vi "Albert_Arr_QueryString.vi"(10 "字符串":string, 11 "2D Arr Input":string[][](array[string])) -> (3 "2D Arr Output":string[][](array[string]))   [LabVIEW 2018]
panel:
  out "数值":i32
  out "布尔":bool=TRUE
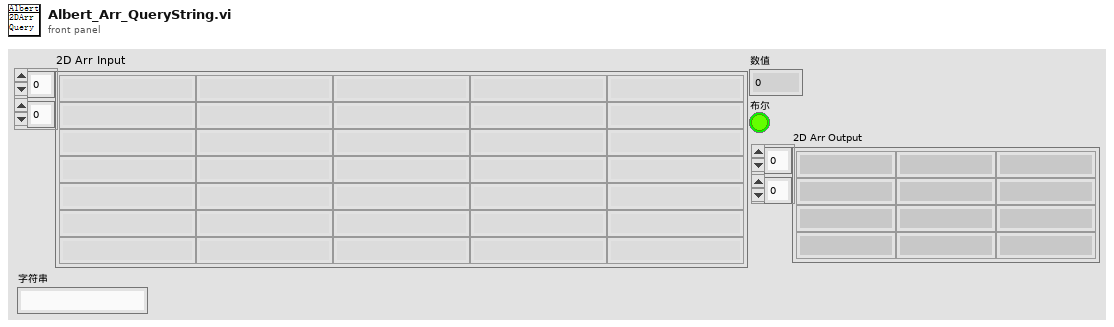
[diagram p1: front panel]
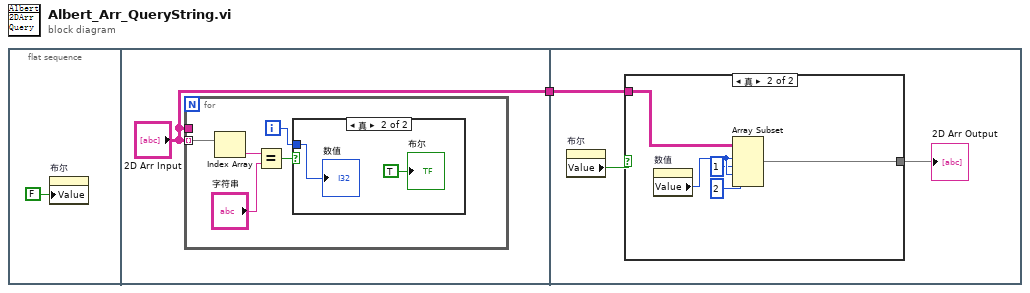
[diagram p0: block diagram]
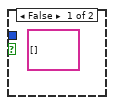
[diagram p2: hidden frame]
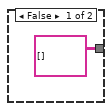
[diagram p3: hidden frame]
diagram:
  n1 = flat-sequence {
    tunnel: ["2D Arr Input"] -> w1
    tunnel: w1 -> [w13]
    frame #0 {
      n2 = property on="布尔" class="Bool (严格)"("Value"=FALSE ("布尔")) -> ()  [unwired: 2 in, 2 out]
    }
    frame #1 {
      n3 = for {
        tunnel: "2D Arr Input" -> [w8] mode=indexing
        tunnel: "2D Arr Input" -> [_]
        i -> [w4]
        n4 = Index Array(array=w8) -> (element=w7:string)  [unwired: 1 in]
        n5 = Equal?(x=w7, y="字符串") -> (x = y?=w5:bool)
        n6 = case shown="真" w5 {
          tunnel: w4 -> [_ w10]
          frame False {
            (unwired) string[][] []
          }
          frame True {
            "数值" <- w10
            "布尔" <- TRUE
          }
        }
      }
    }
    frame #2 {
      n7 = property on="布尔" class="Bool (严格)"() -> ("Value"=w12:bool)  [unwired: 2 in, 2 out]
      n8 = case shown="真" w12 {
        tunnel: w13 -> [_ w19]
        tunnel: [string[][] [] w15] -> w11
        frame False {
        }
        frame True {
          n9 = property on="数值" class="DigNum (严格)"() -> ("Value"=w18:i32)  [unwired: 2 in, 2 out]
          n10 = Array Subset(array=w19, index (row)=w18, length (row)=1 ("长度"), index (col)=w18, length (col)=2 ("长度")) -> (w15:string[][])
        }
      }
      "2D Arr Output" <- w11
    }
  }
